vi "PicoErrorHandler2.vi"(8 "error in (no error)":errorcluster, 10 "Default handle":i16=16384, 11 "handle In":i16=16384) -> (0 "error out":errorcluster)   [LabVIEW 2020]
doc: "This VI takes an error cluster and if an error has occurred, displays a message box indicating the source of the error and the status code returned by the driver."
uses:
  ps3000a.dll
  ps4000a.dll
  ps5000a.dll
  ps6000.dll
  ps2000.dll
  ps4000.dll
  ps5000.dll
  ps3000.dll
  ps2000a.dll
  ps6000a.dll
panel:
  out "CloseUnit Statuses":T1
  out "Pass or Unknown string":string
  out "Error String":string
  out "handle out":i16=16384
  in  "no error":errorcluster
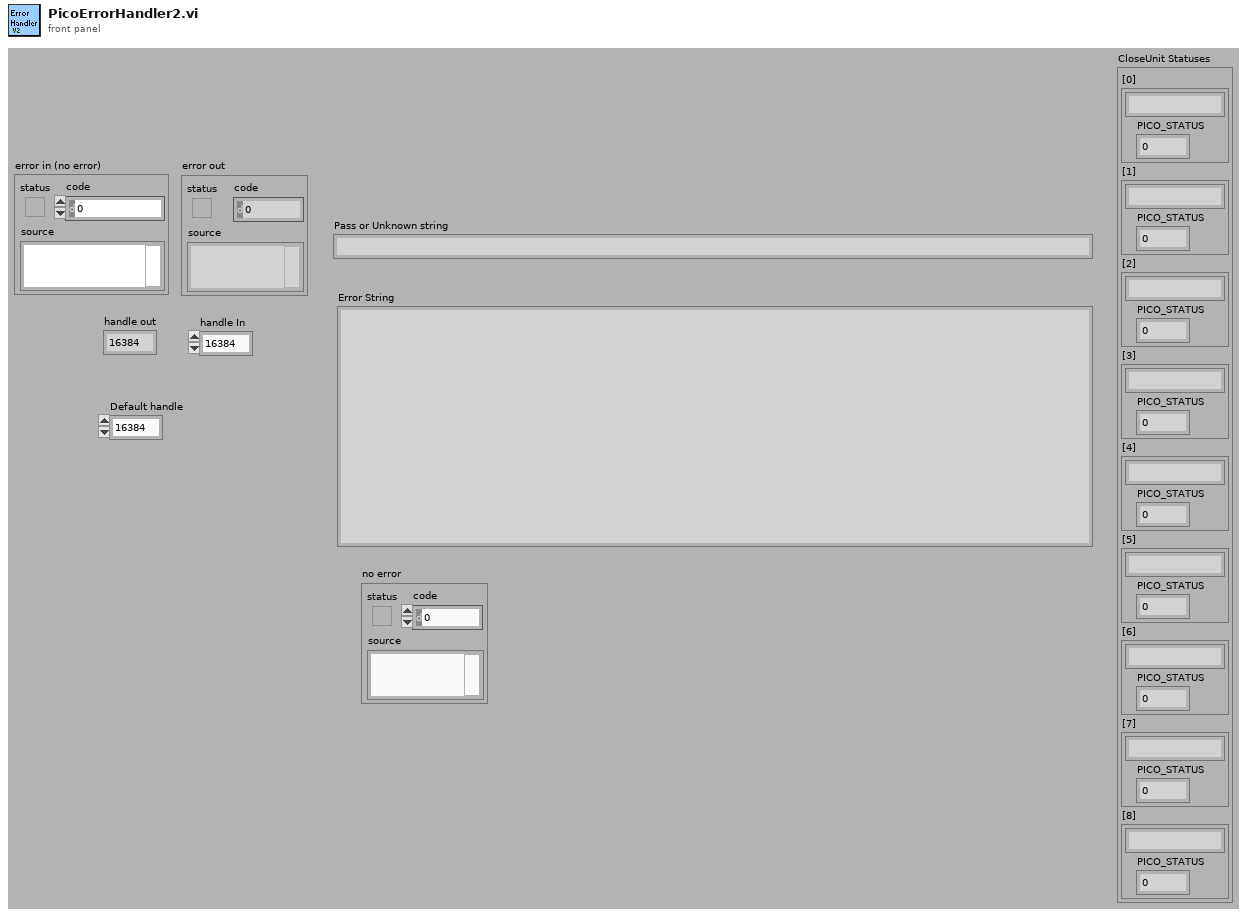
[diagram p1: front panel]
types:
  T1 = cluster{"[0]":cluster{string, "PICO_STATUS":u32}, "[1]":cluster{string, "PICO_STATUS":u32}, "[2]":cluster{string, "PICO_STATUS":u32}, "[3]":cluster{string, "PICO_STATUS":u32}, "[4]":cluster{string, "PICO_STATUS":u32}, "[5]":cluster{string, "PICO_STATUS":u32}, "[6]":cluster{string, "PICO_STATUS":u32}, "[7]":cluster{string, "PICO_STATUS":u32}, "[8]":cluster{string, "PICO_STATUS":u32}}
  T2 = enum16{"Left Button", "Center Button", "Right Button", "Window Close"}
  T3 = cluster{"[0]":cluster{"source":string, "PICO_STATUS":u32}, "[1]":cluster{"source":string, "PICO_STATUS":u32}, "[2]":cluster{"source":string, "PICO_STATUS":u32}, "[3]":cluster{"source":string, "PICO_STATUS":u32}, "[4]":cluster{"source":string, "PICO_STATUS":u32}, "[5]":cluster{"source":string, "PICO_STATUS":u32}, "[6]":cluster{"source":string, "PICO_STATUS":u32}, "[7]":cluster{"source":string, "PICO_STATUS":u32}, "[8]":cluster{"source":string, "PICO_STATUS":u32}}
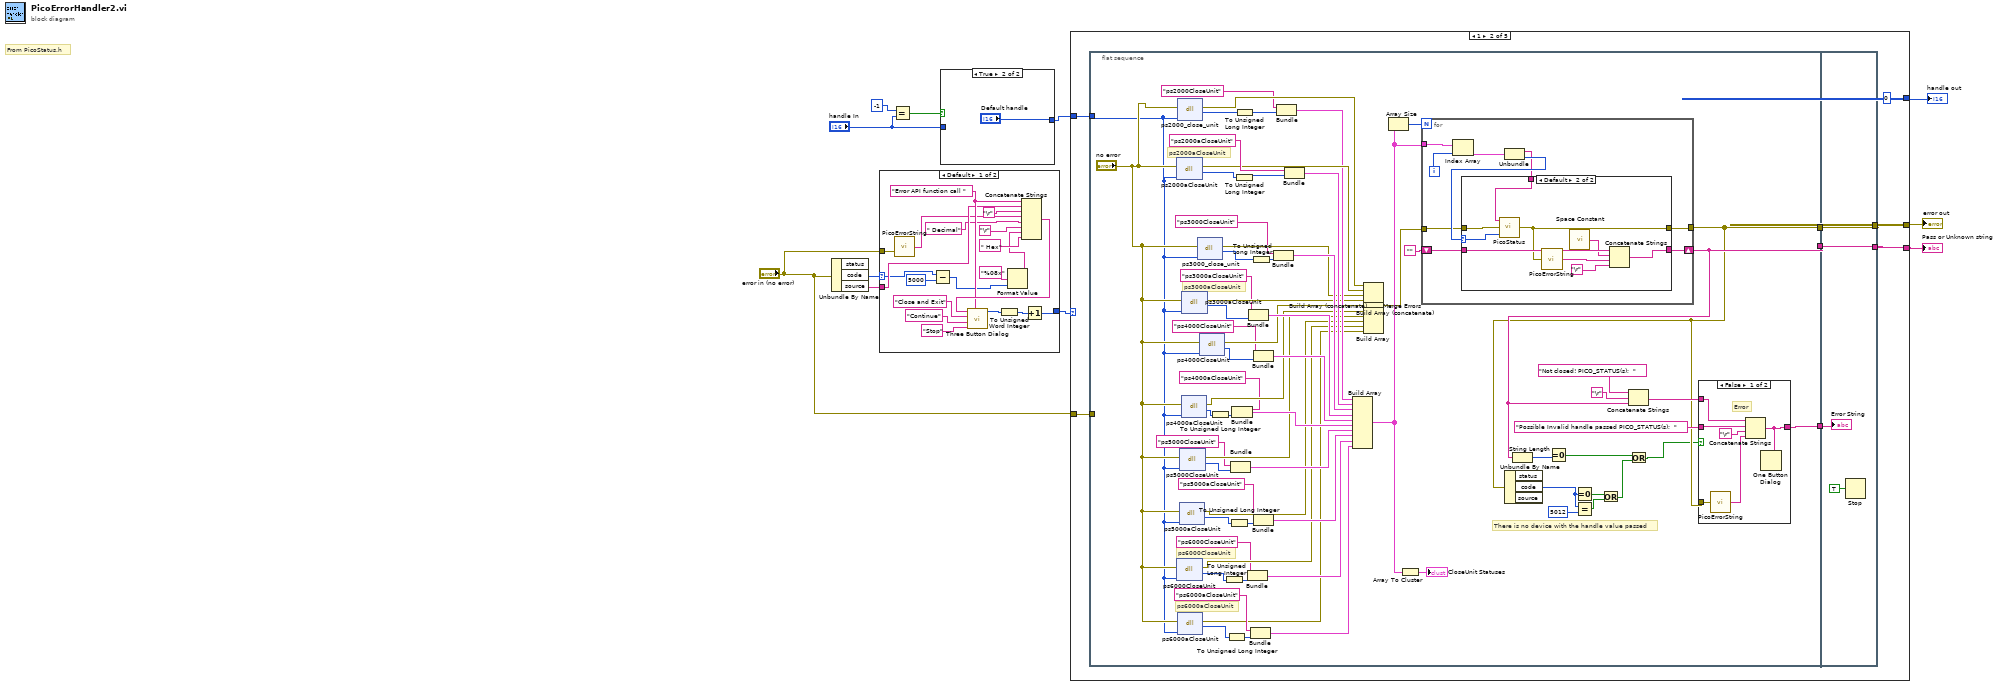
[diagram p0: block diagram]
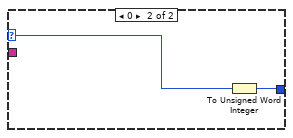
[diagram p3: hidden frame]
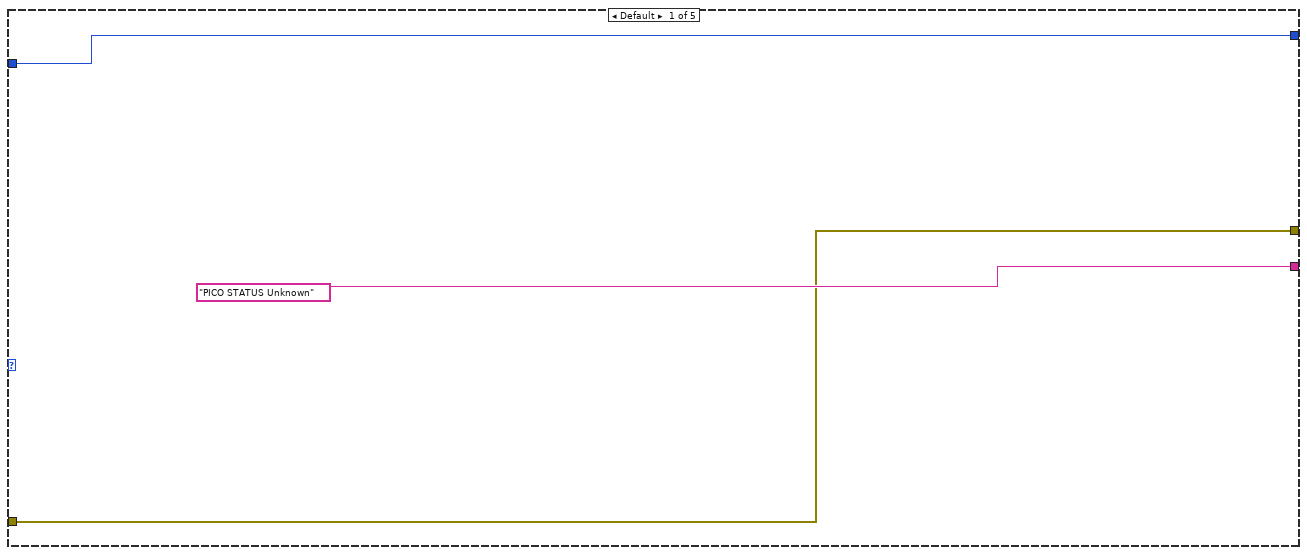
[diagram p4: hidden frame]
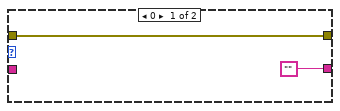
[diagram p6: hidden frame]
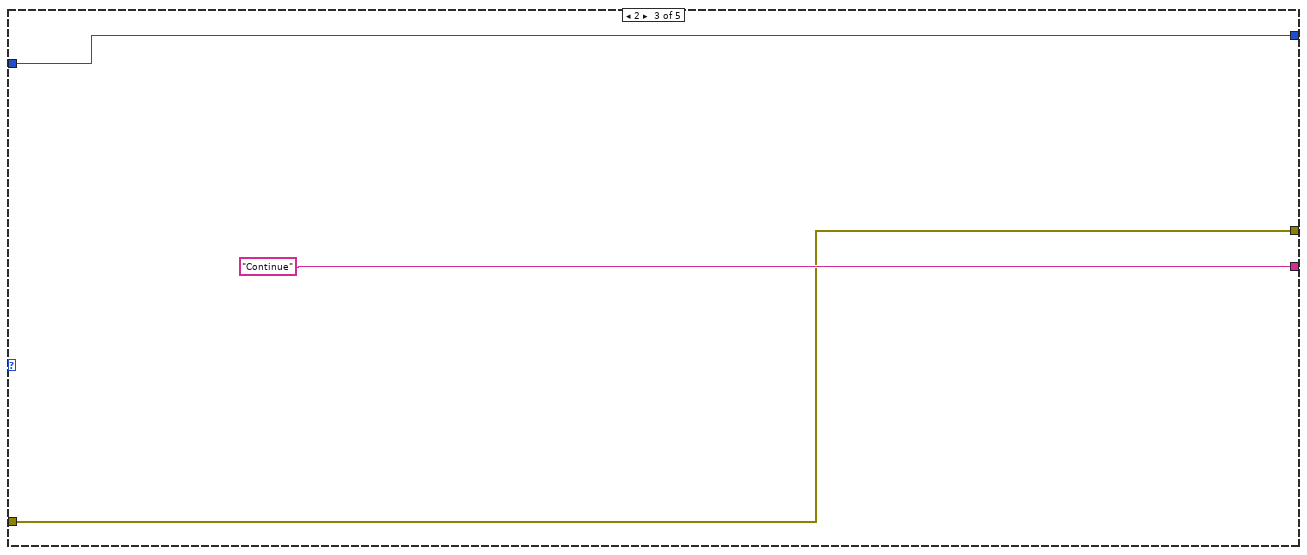
[diagram p7: hidden frame]
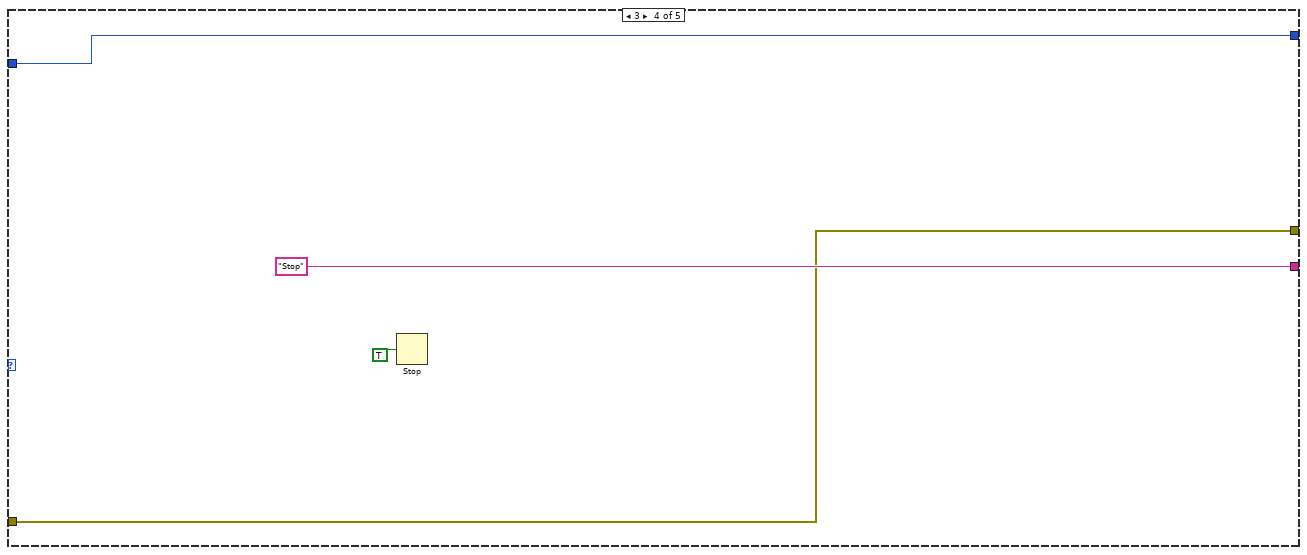
[diagram p8: hidden frame]
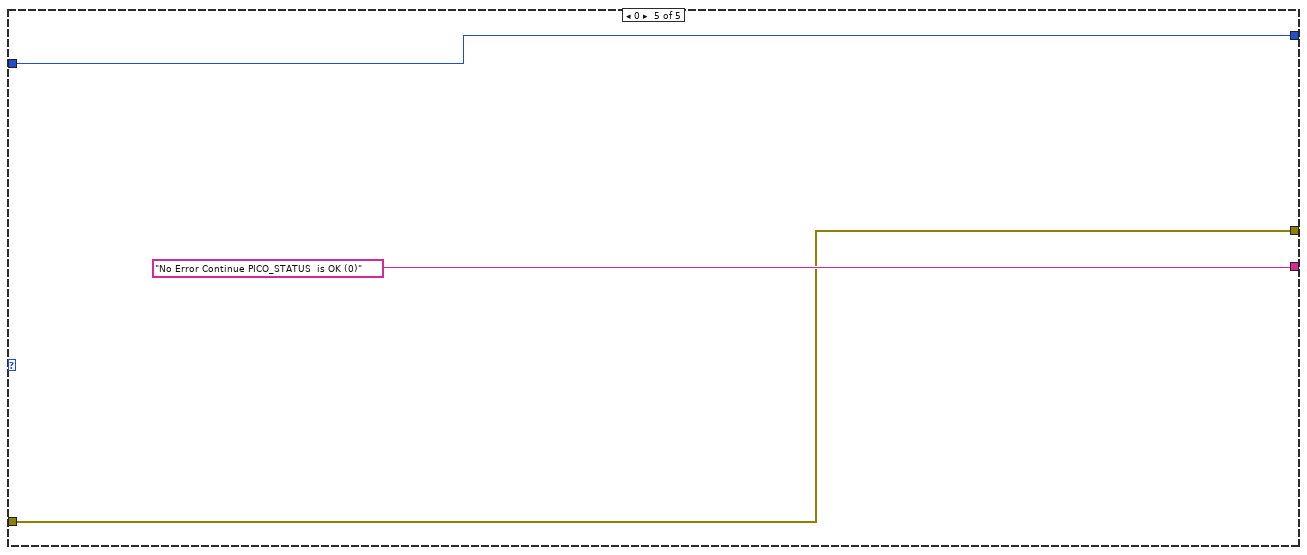
[diagram p9: hidden frame]
diagram:
  # "From PicoStatus.h"
  n1 = Unbundle By Name("error in (no error)") -> ("code"=w10:i32, "source"=w11:string)  [unwired: 1 out]
  n2 = case shown="Default" w10 {
    selector: w10 -> [w16 w32]
    tunnel: w11 -> [w23 _]
    tunnel: [w26 w33] -> w8
    tunnel: "error in (no error)" -> [w21 _]
    frame Default {
      w27 = "Error API function call "
      n3 = call "PicoErrorString.vi"("error in"=w21) -> ("String"=w20:string)  [unwired: 2 in, 2 out]
      n4 = Subtract(x=w16, y=5000) -> (x-y=w19:i32)
      n5 = Format Value(format string="%08x", value (0)=w19) -> (output string=w14:string)  [unwired: 1 in]
      n6 = Concatenate Strings(w27, w23, "\r", w20, " Decimal", "\r", w14, " Hex") -> (w28:string)
      n7 = call "Three Button Dialog.vi"("Window Title (\"\")"=w27, "Right Button Text (\"Cancel\")"="Stop" ("Right Button Text (\"Cancel\")"), "Center Button Text (\"No\")"="Continue" ("Center Button Text (\"No\")"), "Left Button Text (\"Yes\")"="Close and Exit" ("Left Button Text (\"Yes\")"), "message"=w28) -> ("Which Button?"=w24:T2)  [unwired: 6 in]
      n8 = To Unsigned Word Integer(number=w24) -> (unsigned 16bit integer=w25:u16)
      n9 = Increment(x=w25) -> (x+1=w26:u16)
    }
    frame 0 {
      n10 = To Unsigned Word Integer(number=w32) -> (unsigned 16bit integer=w33:u16)
    }
  }
  n11 = Equal?(x=i16 -1, y="handle In") -> (x = y?=w4:bool)
  n12 = case shown="True" w4 {
    tunnel: "handle In" -> [w34 _]
    tunnel: [w34 "Default handle"] -> w2
    frame False {
    }
    frame True {
    }
  }
  n13 = case shown="1" w8 {
    tunnel: w2 -> [w36 w46 w150 w153 w157]
    tunnel: ["PICO STATUS Unknown" w44 "Continue" ("Center Button Text (\"No\")") "Stop" ("Right Button Text (\"Cancel\")") "No Error Continue PICO_STATUS  is OK (0)" ("Center Button Text (\"No\")")] -> w6
    tunnel: [w37 w43 w151 w155 w158] -> w9
    tunnel: "error in (no error)" -> [w37 w45 w151 w155 w158]
    tunnel: [w36 i16 0 ("handle In") w150 w153 w157] -> w7
    frame Default {
    }
    frame 1 {
      n14 = flat-sequence {
        tunnel: w46 -> [w50]
        tunnel: w45 -> [_]
        tunnel: [w111] -> w42
        tunnel: [w60] -> w41
        tunnel: [w109] -> w40
        tunnel: [w148] -> w43
        tunnel: [w149] -> w44
        tunnel: w42 -> [w149]
        tunnel: w41 -> [w148]
        tunnel: w40 -> [w146]
        frame #0 {
          # "ps6000aCloseUnit"
          # "ps6000CloseUnit"
          # "ps3000aCloseUnit"
          # "There is no device with the handle value passed"
          # "ps2000aCloseUnit"
          n15 = dll-call lib="ps2000a.dll" fn="ps2000aCloseUnit" ("ps3000.dll:_ps3000_open_unit@0")(error in="no error", "handle"=w50) -> (error out=w115:errorcluster, "PICO_STATUS"=w87:i32)  [unwired: 3 in, 1 out]
          n16 = dll-call lib="PS6000.dll" fn="ps6000CloseUnit" ("ps3000.dll:_ps3000_open_unit@0")(error in="no error", "handle"=w50) -> (error out=w90:errorcluster, "PICO_STATUS"=w65:i32)  [unwired: 3 in, 1 out]
          n17 = dll-call lib="ps2000.dll" fn="ps2000_close_unit"(error in="no error", "handle"=w50) -> (error out=w86:errorcluster, "return"=w79:i16)  [unwired: 3 in, 1 out]
          n18 = dll-call lib="ps6000a.dll" fn="ps6000aCloseUnit"(error in="no error", "handle"=w50) -> (error out=w48:errorcluster, "PICO_STATUS"=w52:u32)  [unwired: 3 in, 1 out]
          n19 = dll-call lib="ps5000a.dll" fn="ps5000aCloseUnit" ("ps3000.dll:_ps3000_open_unit@0")(error in="no error", "handle"=w50) -> (error out=w91:errorcluster, "PICO_STATUS"=w63:i32)  [unwired: 3 in, 1 out]
          n20 = dll-call lib="PS5000.dll" fn="ps5000CloseUnit" ("ps3000.dll:_ps3000_open_unit@0")(error in="no error", "handle"=w50) -> (error out=w92:errorcluster, "PICO_STATUS"=w69:u32)  [unwired: 3 in, 1 out]
          n21 = dll-call lib="ps4000a.dll" fn="ps4000aCloseUnit" ("ps3000.dll:_ps3000_open_unit@0")(error in="no error", "handle"=w50) -> (error out=w93:errorcluster, "PICO_STATUS"=w61:i32)  [unwired: 3 in, 1 out]
          n22 = dll-call lib="ps3000a.dll" fn="ps3000aCloseUnit" ("ps3000.dll:_ps3000_open_unit@0")(error in="no error", "handle"=w50) -> (error out=w95:errorcluster, "PICO_STATUS"=w78:u32)  [unwired: 3 in, 1 out]
          n23 = dll-call lib="ps3000.dll" fn="ps3000_close_unit" label="CloseUnit"(error in="no error", "handle"=w50) -> (error out=w96:errorcluster, "status"=w67:i16)  [unwired: 3 in, 1 out]
          n24 = dll-call lib="ps4000.dll" fn="ps4000CloseUnit" ("ps3000.dll:_ps3000_open_unit@0")(error in="no error", "handle"=w50) -> (error out=w94:errorcluster, "PICO_STATUS"=w71:u32)  [unwired: 3 in, 1 out]
          n25 = To Unsigned Long Integer(number=w61) -> (unsigned 32bit integer=w62:u32)
          n26 = To Unsigned Long Integer(number=w65) -> (unsigned 32bit integer=w66:u32)
          n27 = To Unsigned Long Integer(number=w52) -> (unsigned 32bit integer=w54:u32)
          n28 = To Unsigned Long Integer(number=w63) -> (unsigned 32bit integer=w64:u32)
          n29 = Bundle("ps5000CloseUnit", "PICO_STATUS"=w69) -> (w100:cluster{string, "PICO_STATUS":u32})  [unwired: 1 in]
          n30 = Bundle("ps4000aCloseUnit", w62) -> (w101:cluster{string, u32})  [unwired: 1 in]
          n31 = To Unsigned Long Integer(number=w87) -> (unsigned 32bit integer=w88:u32)
          n32 = To Unsigned Long Integer(number=w79) -> (unsigned 32bit integer=w80:u32)
          n33 = Bundle("ps6000CloseUnit", w66) -> (w98:cluster{string, u32})  [unwired: 1 in]
          n34 = Bundle("ps3000aCloseUnit", "PICO_STATUS"=w78) -> (w103:cluster{string, "PICO_STATUS":u32})  [unwired: 1 in]
          n35 = Bundle("source"="ps6000aCloseUnit", w54) -> (w49:cluster{"source":string, u32})  [unwired: 1 in]
          n36 = To Unsigned Long Integer(number=w67) -> (unsigned 32bit integer=w68:u32)
          n37 = Bundle("ps4000CloseUnit", "PICO_STATUS"=w71) -> (w102:cluster{string, "PICO_STATUS":u32})  [unwired: 1 in]
          n38 = Bundle("ps5000aCloseUnit", w64) -> (w99:cluster{string, u32})  [unwired: 1 in]
          n39 = Bundle("ps3000CloseUnit", w68) -> (w104:cluster{string, u32})  [unwired: 1 in]
          n40 = Bundle("ps2000CloseUnit", w80) -> (w106:cluster{string, u32})  [unwired: 1 in]
          n41 = Bundle("ps2000aCloseUnit", w88) -> (w105:cluster{string, u32})  [unwired: 1 in]
          n42 = Build Array(w106, w105, w104, w103, w102, w101, w100, w99, w98, w49) -> (w117:cluster{"source":string, "PICO_STATUS":u32}[])
          n43 = Build Array(w86, w115, w96, w95, w94, w93, w92, w91, w90, w48) -> (w59:errorcluster[])
          n44 = Build Array (concatenate)(w59) -> (w55:errorcluster[])
          n45 = Build Array (concatenate)(w55) -> (w47:errorcluster[])
          n46 = Merge Errors(w47) -> (w114:errorcluster)
          n47 = Array Size(array=w117) -> (size(s)=w89:i32)
          n48 = Array To Cluster(array=w117) -> (cluster=→"CloseUnit Statuses":T3)
          n49 = for {
            N: w89 -> [_]
            shift-right: [w129] -> w111
            shift-left: "" -> [w130]
            tunnel: w117 -> [w134]
            tunnel: w114 -> [w128]
            tunnel: [w127] -> w60
            i -> [w133]
            n50 = Index Array(array=w134, index=w133) -> (element=w132:cluster{"source":string, "PICO_STATUS":u32})
            n51 = Unbundle(w132) -> ("source"=w126:string, "PICO_STATUS"=w131:u32)
            n52 = case shown="Default" w131 {
              selector: w131 -> [_ w144]
              tunnel: ["" w145] -> w129
              tunnel: w130 -> [_ w143]
              tunnel: w128 -> [w135 w139]
              tunnel: [w135 w138] -> w127
              tunnel: w126 -> [_ w137]
              frame 0 {
              }
              frame Default {
                n53 = call "PicoStatus.vi"("PICO STATUS"=w144, "error in"=w139, "source"=w137) -> ("error out"=w138:errorcluster)
                n54 = call "PicoErrorString.vi"("error in"=w138) -> ("String"=w141:string)  [unwired: 2 in, 2 out]
                n55 = call "Space Constant.vi"() -> ("String"=w142:string)
                n56 = Concatenate Strings(w143, w142, w141, "\r") -> (w145:string)
              }
            }
          }
          n57 = Unbundle By Name(w60) -> ("code"=w82:i32)  [unwired: 2 out]
          n58 = String Length(string=w111) -> (length=w110:i32)
          n59 = Equal To 0?(x=w110) -> (x = 0?=w57:bool)
          n60 = Equal To 0?(x=w82) -> (x = 0?=w85:bool)
          n61 = Equal?(x=w82, y=5012) -> (x = y?=w84:bool)
          n62 = Or(x=w85, y=w84) -> (x .or. y?=w58:bool)
          n63 = Concatenate Strings("Not closed! PICO_STATUS(s);  " ("Left Button Text (\"Yes\")"), "\r", w111) -> (w108:string)
          n64 = Or(x=w57, y=w58) -> (x .or. y?=w56:bool)
          n65 = case shown="False" w56 {
            tunnel: [w119 w125] -> w109
            tunnel: w108 -> [w123 w125]
            tunnel: "Possible Invalid handle passed PICO_STATUS(s);  " ("Left Button Text (\"Yes\")") -> [w122 _]
            tunnel: w60 -> [w121 _]
            frame False {
              # "Error"
              n66 = call "PicoErrorString.vi"("error in"=w121) -> ("String"=w120:string)  [unwired: 2 in, 2 out]
              n67 = Concatenate Strings(w123, w122, "\r", w120) -> (w119:string)
              n68 = One Button Dialog(message=w119) -> ()  [unwired: 1 in, 1 out]
            }
            frame True {
            }
          }
        }
        frame #1 {
          n69 = Stop(stop? (T)=TRUE) -> ()
          "Error String" <- w146
        }
      }
    }
    frame 2 {
    }
    frame 3 {
      n70 = Stop(stop? (T)=TRUE) -> ()
    }
    frame 0 {
    }
  }
  "error out" <- w9
  "handle out" <- w7
  "Pass or Unknown string" <- w6
